vi "Not a Number.vi"(1 "Input":dbl) -> (0 "Output":dbl)   [LabVIEW 2014]
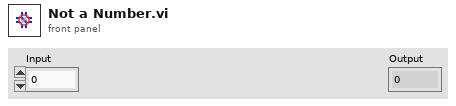
[diagram p1: front panel]
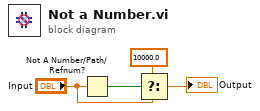
[diagram p0: block diagram]
diagram:
  n1 = Not A Number/Path/Refnum?(number/path/refnum="Input") -> (NaN/Path/Refnum?=w4:bool)
  n2 = Select(t=10000.0, s=w4, f="Input") -> (s? t:f=→"Output":dbl)
